vi "Get logging.vi"(8 "error in (no error)":errorcluster, 11 "Piezo in":refnum<class "Piezo.lvclass">) -> (0 "error out":errorcluster, 2 "logging?":bool, 3 "Piezo out":refnum<class "Piezo.lvclass">)   [LabVIEW 2012, in "Piezo.lvclass"]
uses:
  Piezo.lvclass
  Piezo.lvclass/Piezo.ctl
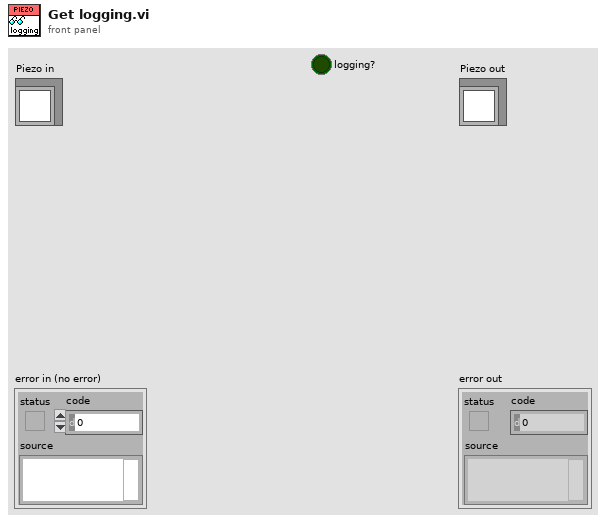
[diagram p1: front panel]
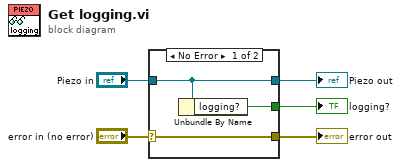
[diagram p0: block diagram]
diagram:
  n1 = case shown="No Error" "error in (no error)" {
    selector: "error in (no error)" -> [w8 w10]
    tunnel: [w8 w10] -> w4
    tunnel: [w7 w9] -> w2
    tunnel: "Piezo in" -> [w7 w9]
    tunnel: [w6 _] -> w1
    frame No Error {
      n2 = Unbundle By Name(w7) -> ("logging?"=w6:bool)
    }
    frame Error {
    }
  }
  "error out" <- w4
  "Piezo out" <- w2
  "logging?" <- w1
